vi "initialize.vi"(8 "error in (no error)":errorcluster, 10 "MCListbox Refnum":refnum<vi>, 11 "AbstractMultiColumnListBoxAdapter in":refnum<class "AbstractMultiColumnListBoxAdapter.lvclass">) -> (0 "error out":errorcluster, 3 "AbstractMultiColumnListBoxAdapter out":refnum<class "AbstractMultiColumnListBoxAdapter.lvclass">)   [LabVIEW 2020, in "AbstractMultiColumnListBoxAdapter.lvclass"]
uses:
  AbstractMultiColumnListBoxAdapter.lvclass
  AbstractMultiColumnListBoxAdapter.lvclass/AbstractMultiColumnListBoxAdapter.ctl
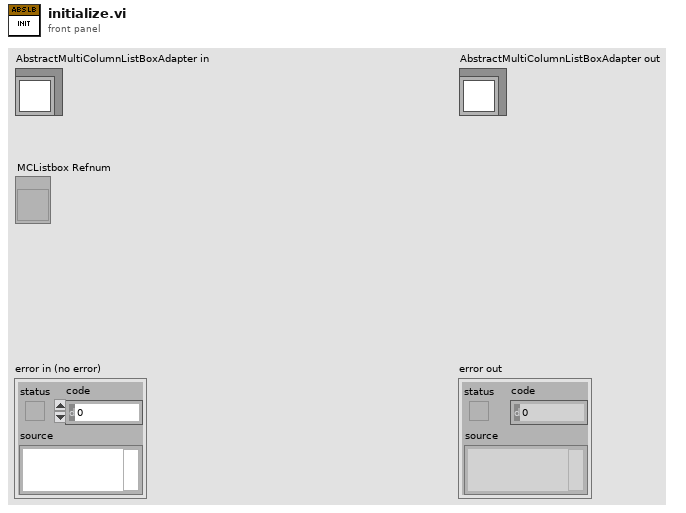
[diagram p1: front panel]
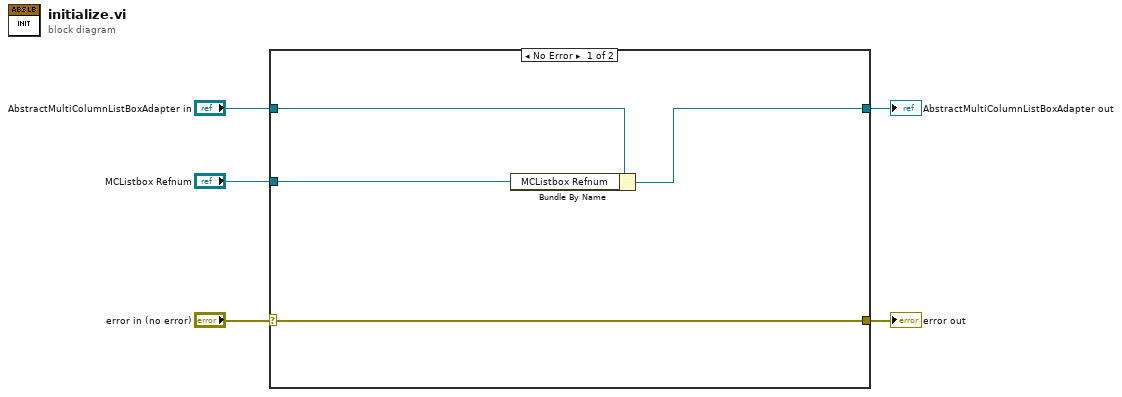
[diagram p0: block diagram]
diagram:
  n1 = case shown="No Error" "error in (no error)" {
    selector: "error in (no error)" -> [w9 w11]
    tunnel: [w9 w11] -> w4
    tunnel: [w7 w10] -> w2
    tunnel: "AbstractMultiColumnListBoxAdapter in" -> [w8 w10]
    tunnel: "MCListbox Refnum" -> [w6 _]
    frame No Error {
      n2 = Bundle By Name(cluster=w8, "MCListbox Refnum"=w6) -> (w7:refnum<class "AbstractMultiColumnListBoxAdapter.lvclass">)
    }
    frame Error {
    }
  }
  "error out" <- w4
  "AbstractMultiColumnListBoxAdapter out" <- w2
